vi "Data_File_Init.vi"(0 "Data File Directory":path=path "c:/data", 5 "Test_Name In:":string(combo)="HeatUP", 7 "Version In:":string="DGnn", 9 "Computer Name In:":string="1A", 11 "error in (no error)":errorcluster, 12 "File Extension:":string=".tmp", 13 "Ambient Temp / RH:":string="068,50", 14 "Mode:":string(combo)) -> (4 "FileName":path, 6 "Data Array":string[][](array[string]), 15 "error out":errorcluster)   [LabVIEW 2014]
uses:
  <vilib>/Utility/error.llb/whitespace.ctl
  Type Definitions/HEWH Error Enumeration.ctl
  Global HEWH.vi
  <vilib>/Utility/file.llb/Write To Spreadsheet File (string).vi
panel:
  out "length":i32
  out "Filename":string
  in  "Config File Path":path=path "C:/work/flowconfig.ini"
  in  "Test Number*:":string="001"
  in  "TR Number*:":string="T12345678"
  in  "Unit*:":string="DGnn"
  out "Computer:":string="1A"
  in  "stop":bool
  in  "Comments:":string="R134A Charge Level: 50g"
  in  "Technician:":string="RonR."
  in  "Engineer:":string="CraigT."
  in  "Test Station:":string="0A"
  out "Version:":string="DGnn"
  out "Test_Name*:":string="HeatUP"
  out "Date:":string="DGnn"
  in  "Model*:":string="DGnn"
  # "yyyymmdd_hhmm_ttttt_uuuuuuuuuu_nnn_xx_ppp_Trrrrrrrr\nWhere:\nyyyymmdd - day, month as 3 chars, 4 digit year(automatic)\nhhmm - hour and minute (24 hr) test started (automatic)\nttttt - test type name, (automatic)\nuuuuuuuuu - is unit number\nnnn - First 3 chars of Ambient Temp/RH\nxx - Mode (HY, SE, EH, HD)\nppp - Test Station\nTrrrrrrrr - 8 digit TR #"
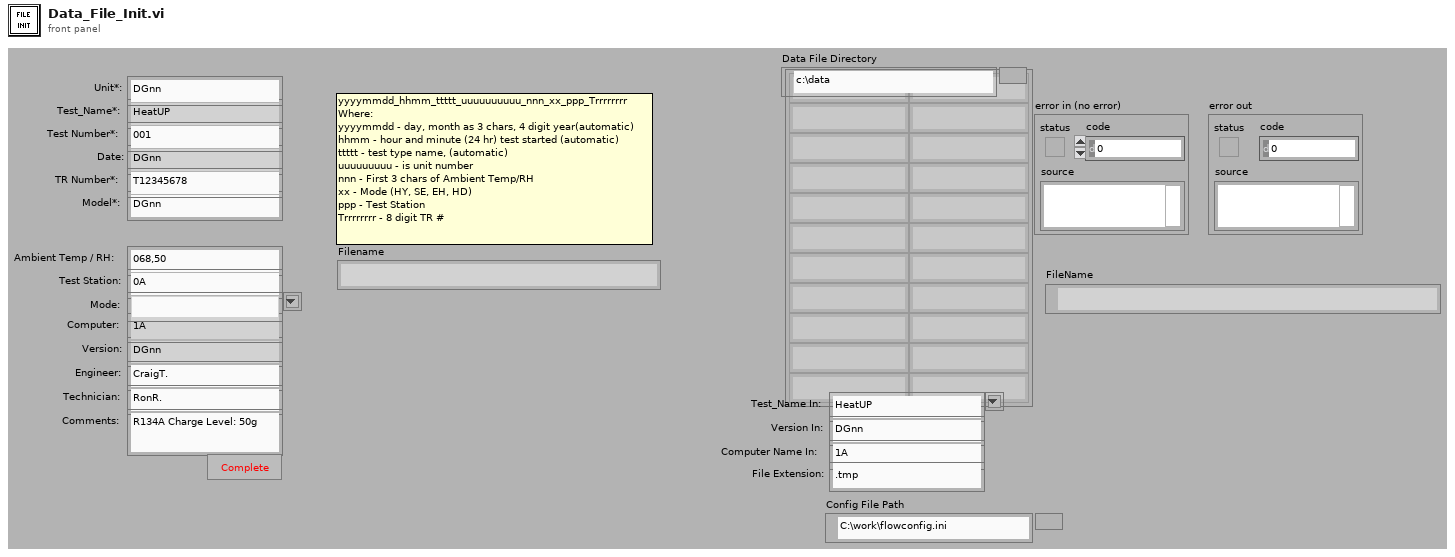
[diagram p1: front panel]
types:
  T1 = typedef "HEWH Error Enumeration.ctl" = enum16{"No Error", "GEA2 Send ACK Mismatch", "GEA2 STX", "GEA2 ETX", "GEA2 CRC Mismatch", "GEA2 ReadACK", "RTD In Range Error", "Fail Mean Tank Temp", "No Flow Config Data Found", "Failed Flow During Purge", "Temp During Purge", "Confirm IF Stop Fail", "Init Draw: TC_1 Out of Range", "Flow = 0 During Draw after 20s"}
  T2 = typedef "whitespace.ctl" = u16
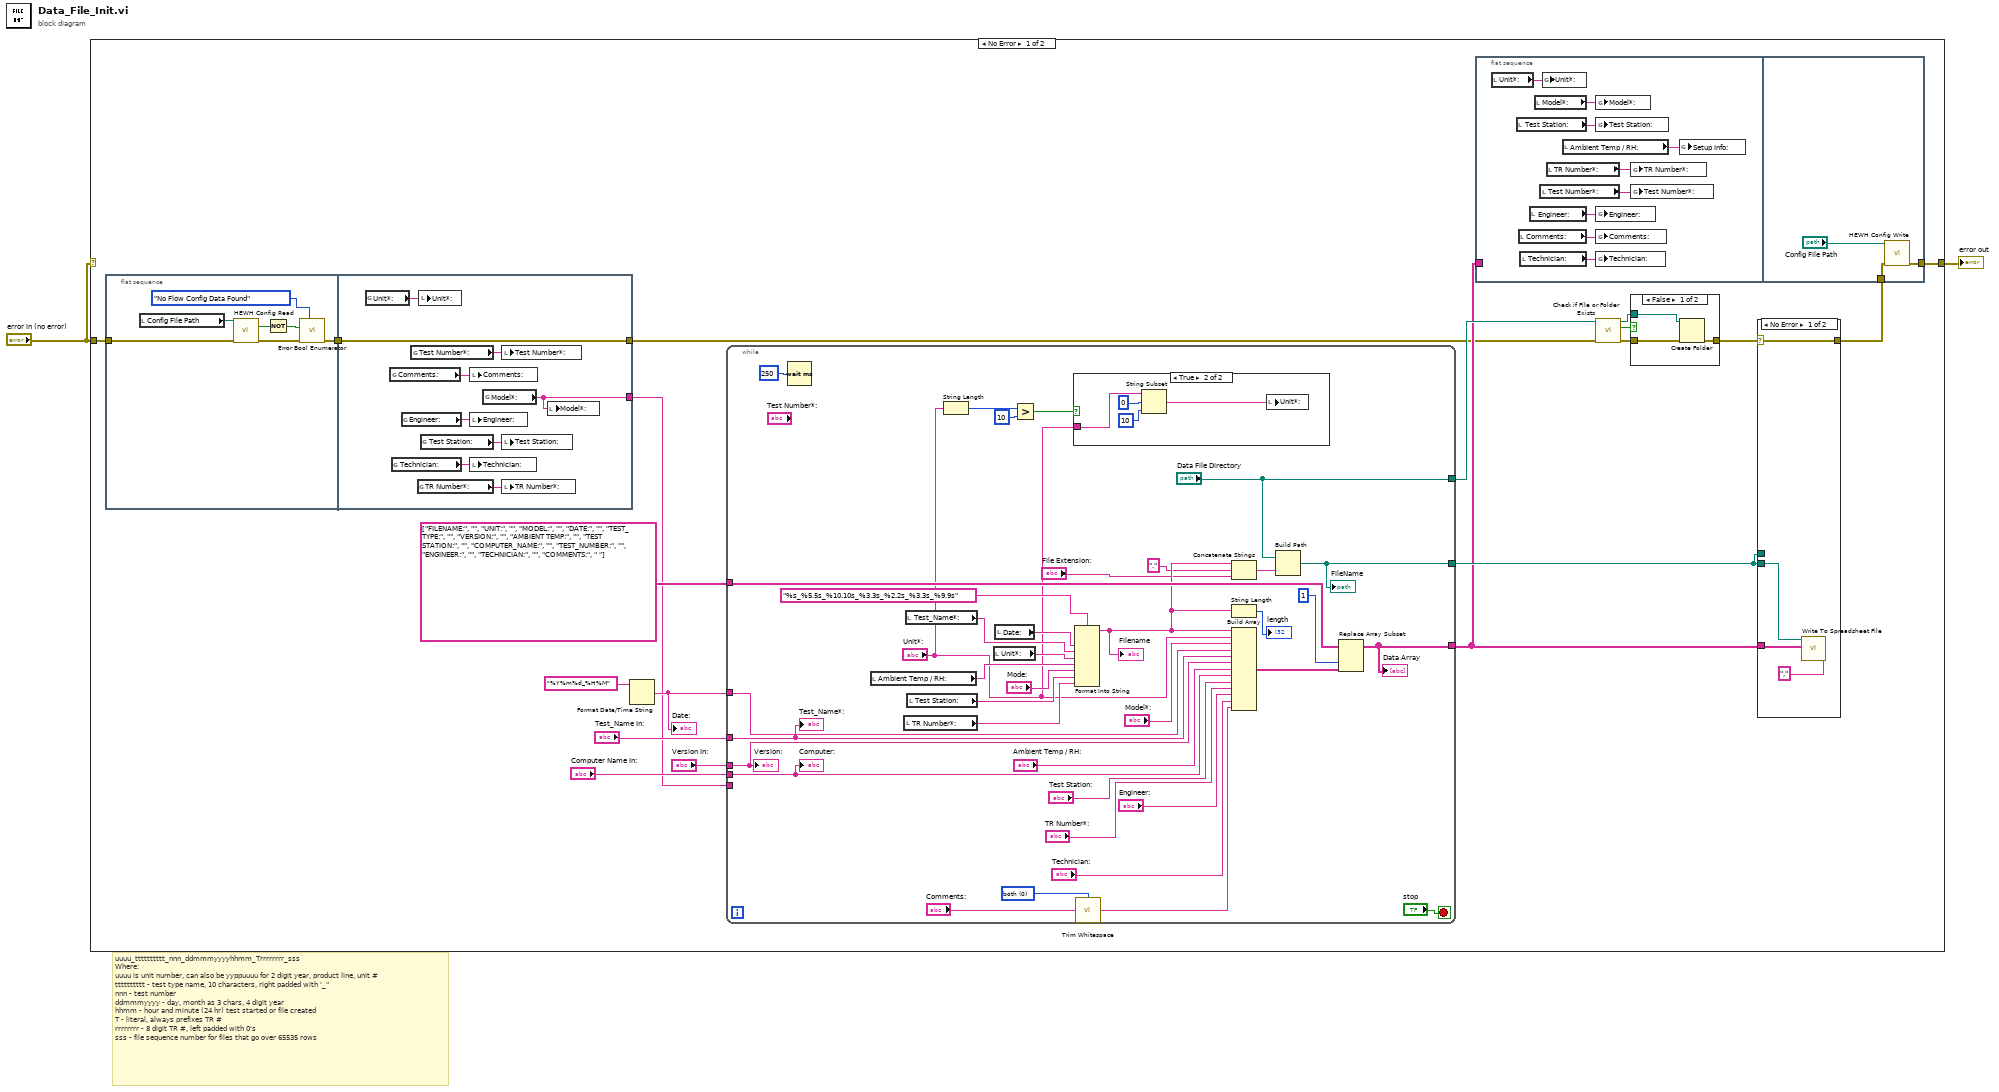
[diagram p0: block diagram]
diagram:
  # "uuuu_tttttttttt_nnn_ddmmmyyyyhhmm_Trrrrrrrr_sss\nWhere:\nuuuu is unit number, can also be yyppuuuu for 2 digit year, product line, unit #\ntttttttttt - test type name, 10 characters, right padded with '_\"\nnnn - test number\nddmmmyyyy - day, month as 3 chars, 4 digit year\nhhmm - hour and minute (24 hr) test started or file created\nT - literal, always prefixes TR #\nrrrrrrrr - 8 digit TR #, left padded with 0's\nsss - file sequence number for files that go over 65535 rows"
  n1 = case shown="No Error" "error in (no error)" {
    selector: "error in (no error)" -> [_ w101]
    tunnel: [w6 w101] -> w2
    tunnel: "error in (no error)" -> [w4 _]
    frame No Error {
      n2 = flat-sequence {
        tunnel: w4 -> [w36]
        tunnel: [w35] -> w21
        tunnel: [w43] -> w8
        tunnel: [w41] -> w3
        tunnel: w21 -> [w41]
        frame #0 {
          n3 = local read "Config File Path"() -> (w34:path)
          n4 = call "HEWH Config Read.vi"("Config File Path"=w34, "error in (no error)"=w36) -> ("found?"=w37:bool, "error out"=w39:errorcluster)  [unwired: 12 in]
          n5 = Not(x=w37) -> (.not. x?=w38:bool)
          n6 = call "Error Bool Enumerator.vi"("Error Enum"=HEWH_Error_Enumeration."No Flow Config Data Found", "Error In"=w39, "Error?"=w38) -> ("Error Out"=w35:errorcluster)  [unwired: 6 in]
        }
        frame #1 {
          n7 = global read "Global HEWH.vi" "Unit*:"() -> (w49:string)
          n8 = global read "Global HEWH.vi" "Comments:"() -> (w46:string)
          n9 = global read "Global HEWH.vi" "Technician:"() -> (w45:string)
          n10 = global read "Global HEWH.vi" "Engineer:"() -> (w44:string)
          n11 = global read "Global HEWH.vi" "Test Number*:"() -> (w48:string)
          n12 = global read "Global HEWH.vi" "TR Number*:"() -> (w47:string)
          n13 = local write "Unit*:"(w49) -> ()
          n14 = global read "Global HEWH.vi" "Test Station:"() -> (w42:string)
          n15 = local write "Comments:"(w46) -> ()
          n16 = local write "Engineer:"(w44) -> ()
          n17 = local write "Technician:"(w45) -> ()
          n18 = global read "Global HEWH.vi" "Model*:"() -> (w43:string)
          n19 = local write "Test Number*:"(w48) -> ()
          n20 = local write "Test Station:"(w42) -> ()
          n21 = local write "TR Number*:"(w47) -> ()
          n22 = local write "Model*:"(w43) -> ()
        }
      }
      n23 = Format Date/Time String(time format string (%c)="%Y%m%d_%H%M") -> (date/time string=w19:string)  [unwired: 2 out]
      "Date:" <- w19
      n24 = while {
        tunnel: w19 -> [w86]
        tunnel: string[][] [["FILENAME:", ""], ["UNIT:", ""], ["MODEL:", ""], ["DATE:", ""], ["TEST_TYPE:", ""], ["VERSION:", ""], ["AMBIENT TEMP:", ""], ["TEST STATION:", ""], ["COMPUTER_NAME:", ""], ["TEST_NUMBER:", ""], ["ENGINEER:", ""], ["TECHNICIAN:", ""], ["COMMENTS:", " "]] ("array") -> [w95]
        tunnel: [w89] -> w7
        tunnel: [w88] -> w13
        tunnel: ["Data File Directory"] -> w12
        tunnel: "Test_Name In:" -> [w84]
        tunnel: "Version In:" -> [w74]
        tunnel: "Computer Name In:" -> [w83]
        tunnel: w8 -> [_]
        stop <- "stop" stop-if-true
        w59 = T2 0 items=["both", "start of string", "end of string"] ("location (both)")
        n25 = Wait (ms)(milliseconds to wait=u32 250) -> ()  [unwired: 1 out]
        n26 = local read "Ambient Temp / RH:"() -> (w75:string)
        n27 = local read "TR Number*:"() -> (w71:string)
        n28 = local read "Test_Name*:"() -> (w77:string)
        n29 = local read "Test Station:"() -> (w72:string)
        n30 = String Length(string="Unit*:") -> (length=w69:i32)
        n31 = local read "Unit*:"() -> (w76:string)
        n32 = local read "Date:"() -> (w78:string)
        n33 = Greater?(x=w69, y=10) -> (0:w67:bool)
        n34 = case shown="True" w67 {
          tunnel: "Unit*:" -> [_ w100]
          frame False {
          }
          frame True {
            n35 = String Subset(string=w100, offset (0)=0, length (rest)=10 ("length (rest)")) -> (substring=w97:string)
            n36 = local write "Unit*:"(w97) -> ()
          }
        }
        n37 = Format Into String(format string="%s_%5.5s_%10.10s_%3.3s_%2.2s_%3.3s_%9.9s", w78, w77, w76, w75, "Mode:", w72, w71) -> (resulting string=w64:string)  [unwired: 2 in, 1 out]
        "Filename" <- w64
        n38 = call <vilib>:"Trim Whitespace.vi"("string"="Comments:", "location (both)"=w59) -> ("trimmed string"=w60:string)
        n39 = Concatenate Strings(w64, "." ("string"), "File Extension:") -> (w65:string)
        n40 = String Length(string=w64) -> (length=→"length":i32)
        n41 = Build Array(w64, "Unit*:", "Model*:", w86, w84, w74, "Ambient Temp / RH:", w83, "Test Station:", "TR Number*:", "Engineer:", "Technician:", w60) -> (w90:string[])
        n42 = Build Path(base path="Data File Directory", name or relative path=w65) -> (appended path=w88:path)
        "FileName" <- w88
        n43 = Replace Array Subset(array=w95, new element=w90, index (col)=1 ("disabled index (col)")) -> (w89:string[][])  [unwired: 1 in]
        "Data Array" <- w89
        "Test_Name*:" <- w84
        "Version:" <- w74
        "Computer:" <- w83
      }
      n44 = flat-sequence {
        tunnel: w7 -> [_]
        tunnel: [w33] -> w6
        tunnel: w5 -> [w32]
        frame #0 {
          n45 = local read "Unit*:"() -> (w30:string)
          n46 = local read "Test Station:"() -> (w22:string)
          n47 = local read "Comments:"() -> (w27:string)
          n48 = local read "Technician:"() -> (w26:string)
          n49 = local read "Engineer:"() -> (w25:string)
          n50 = local read "Model*:"() -> (w23:string)
          n51 = local read "Test Number*:"() -> (w29:string)
          n52 = global write "Global HEWH.vi" "Unit*:"(w30) -> ()
          n53 = local read "TR Number*:"() -> (w28:string)
          n54 = local read "Ambient Temp / RH:"() -> (w24:string)
          n55 = global write "Global HEWH.vi" "Model*:"(w23) -> ()
          n56 = global write "Global HEWH.vi" "Test Station:"(w22) -> ()
          n57 = global write "Global HEWH.vi" "Engineer:"(w25) -> ()
          n58 = global write "Global HEWH.vi" "Comments:"(w27) -> ()
          n59 = global write "Global HEWH.vi" "Technician:"(w26) -> ()
          n60 = global write "Global HEWH.vi" "TR Number*:"(w28) -> ()
          n61 = global write "Global HEWH.vi" "Test Number*:"(w29) -> ()
          n62 = global write "Global HEWH.vi" "Setup Info:"(w24) -> ()
        }
        frame #1 {
          n63 = call "HEWH Config Write.vi"("Config File Path"="Config File Path", "error in (no error)"=w32) -> ("error out"=w33:errorcluster)  [unwired: 13 in]
        }
      }
      n64 = call <vilib>:"Check if File or Folder Exists.vi"("error in (no error)"=w3, "path"=w12) -> ("error out"=w17:errorcluster, "file or folder exists?"=w15:bool, "dup path"=w16:path)  [unwired: 7 out]
      n65 = case shown="False" w15 {
        tunnel: w16 -> [w55 _]
        tunnel: w17 -> [w57 w58]
        tunnel: [w56 w58] -> w14
        frame False {
          n66 = Create Folder(path (use dialog)=w55, error in=w57) -> (error out=w56:errorcluster)  [unwired: 3 out]
        }
        frame True {
        }
      }
      n67 = case shown="No Error" w14 {
        selector: w14 -> [w51 w54]
        tunnel: w13 -> [_ _]
        tunnel: w7 -> [w53 _]
        tunnel: [w51 w54] -> w5
        tunnel: w13 -> [w50 _]
        frame No Error {
          n68 = call-poly <vilib>:"Write To Spreadsheet File.vi"("delimiter (\\t)"="," ("delimiter (\\t)"), "2D data"=w53, "file path (dialog if empty)"=w50) -> ()  [unwired: 5 in, 1 out]
        }
        frame Error {
        }
      }
    }
    frame Error {
    }
  }
  "error out" <- w2
